vi "Gas Switching Menu Bar.vi"() -> ()   [LabVIEW 2015]
uses:
  <vilib>/Utility/miscctls.llb/LVRowAndColumnTypeDef.ctl
  <vilib>/Utility/file.llb/Read Delimited Spreadsheet (string).vi
panel:
  out "disabled index (col)":i32
  out "Color Box 2":u32(colorbox)
  out "Skip Current Row":bool
  out "Elapsed Time":dbl caption="Elapsed Time (s)"
  in  "stop":bool
  in  "Table Control":string[][](table)=[["1", "1", "13"], ["2", "3", "24"], ["3", "4", "31"], ["4", "2", "19"], ["5", "6", "11"], ["6", "8", "28"], ["7", "3", "17"], ["8", "4", "9"], ["9", "3", "14"], ["10", "7", "41"], ["11", "4", "27"], ["12", "2", "18"], ["13", "1", "19"], ["14", "7", "12"], ["15", "8", "28"], ["16", "5", "18"], ["17", "3", "27"], ["18", "2", "13"], ["19", "1", "31"], ["20", "6", "24"]]
  # "Auto Gas Switching"
  # "seconds"
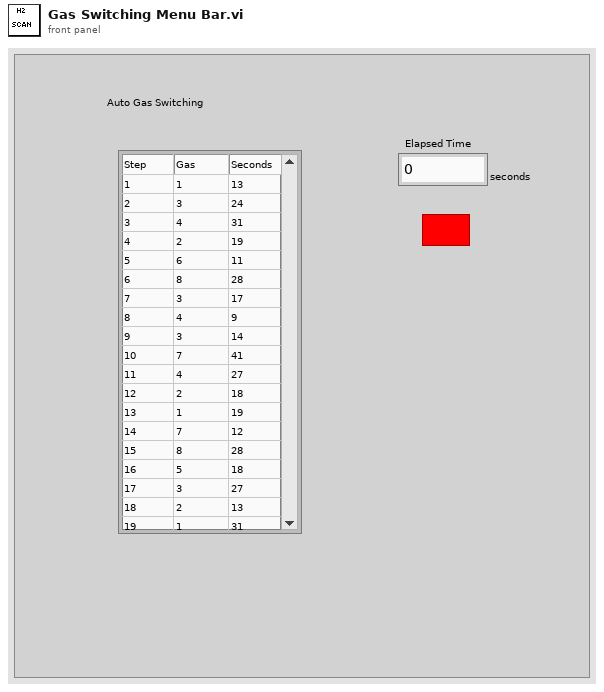
[diagram p1: front panel]
types:
  T1 = typedef "LVRowAndColumnTypeDef.ctl" = cluster{"Row":i32, "Column":i32}
  T2 = typedef "LVBoundsTypeDef.ctl" = cluster{"Width":u32, "Height":u32}
  T3 = typedef "LVPositionTypeDef.ctl" = cluster{"Left":i32, "Top":i32}
  T4 = typedef "LVPoint32TypeDef.ctl" = cluster{"Horizontal":i32, "Vertical":i32}
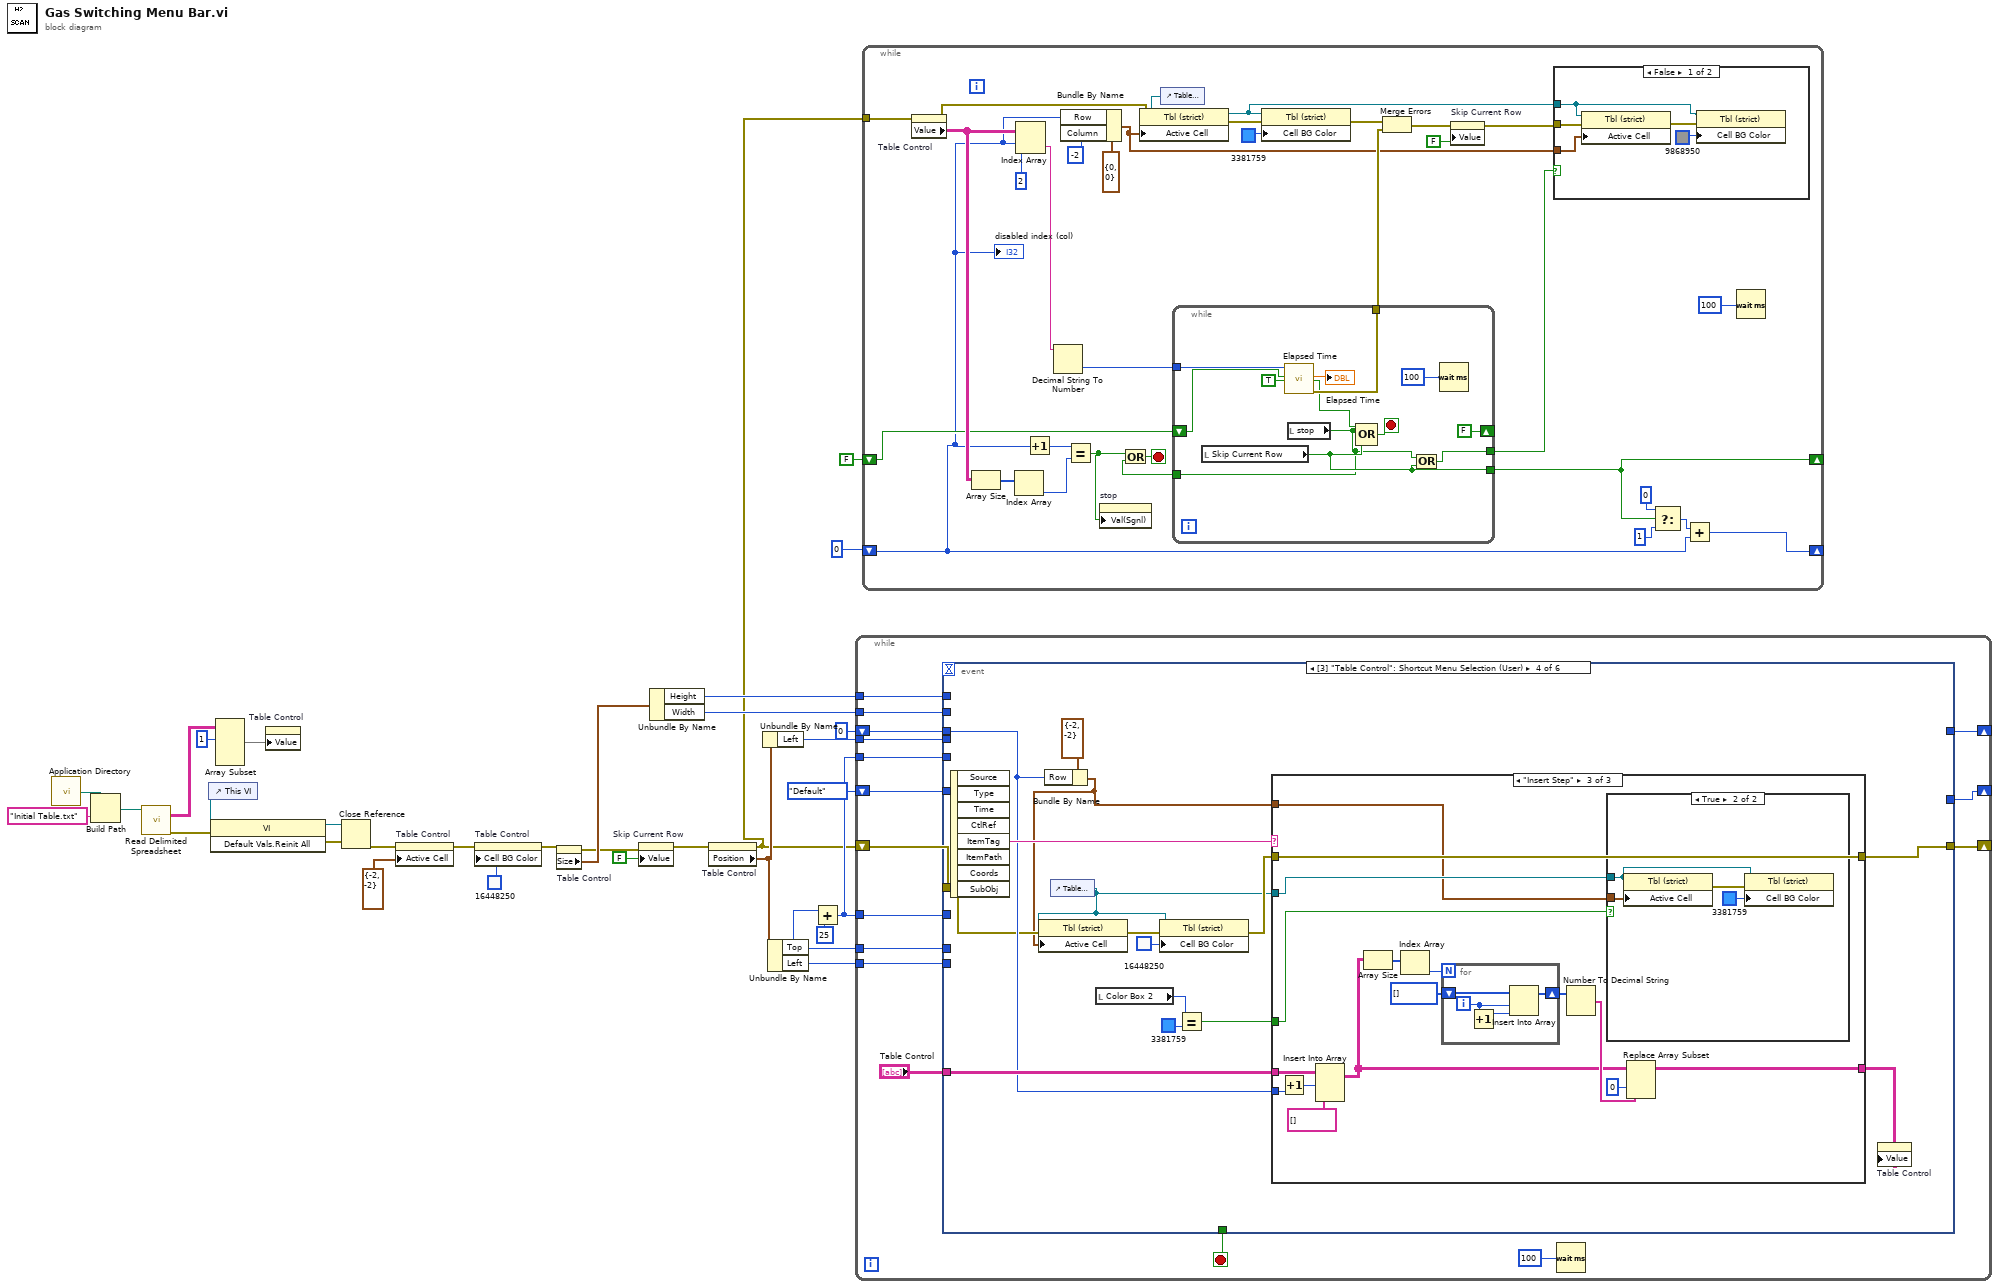
[diagram p0: block diagram]
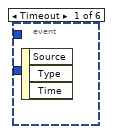
[diagram p3: hidden frame]
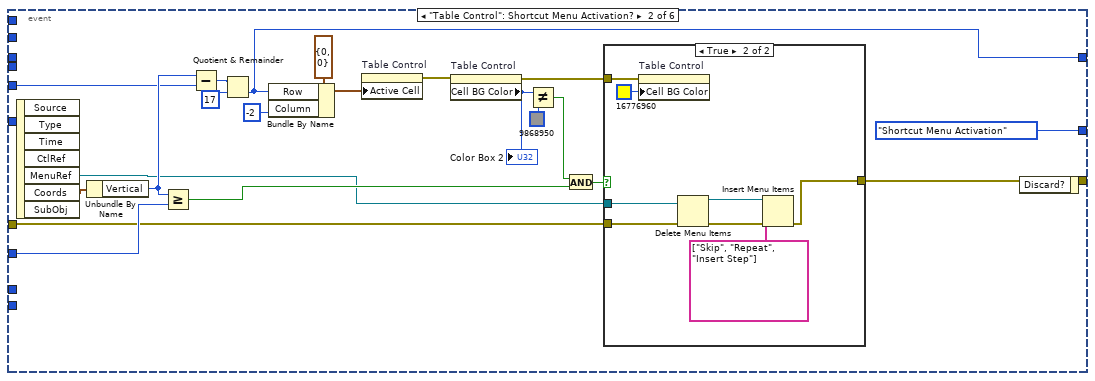
[diagram p4: hidden frame]
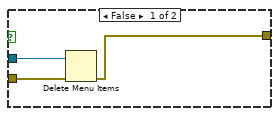
[diagram p5: hidden frame]
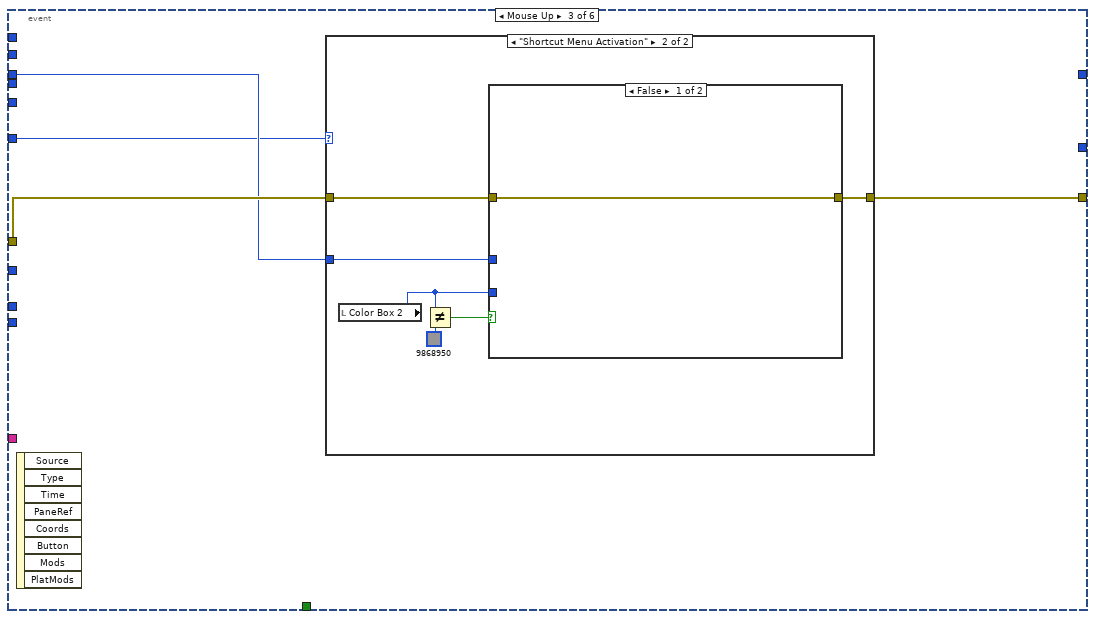
[diagram p6: hidden frame]
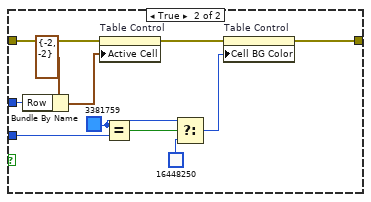
[diagram p8: hidden frame]
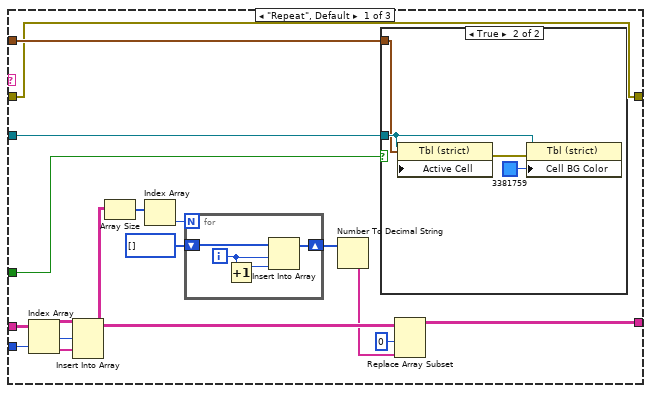
[diagram p9: hidden frame]
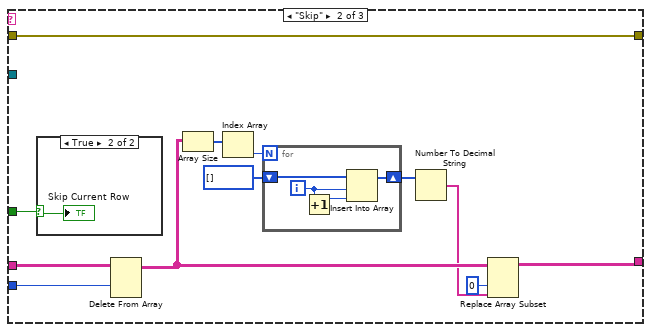
[diagram p11: hidden frame]
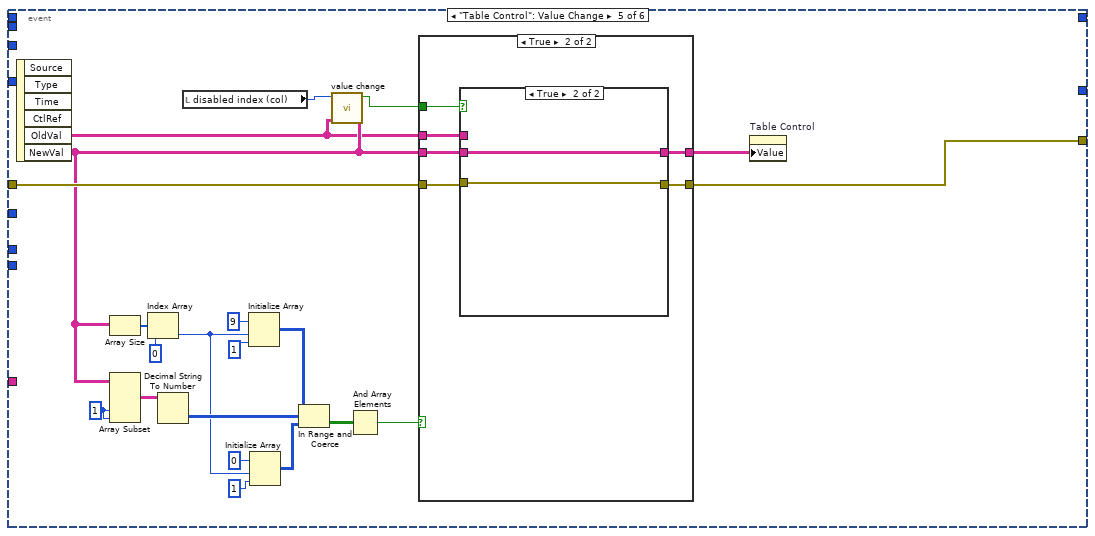
[diagram p14: hidden frame]
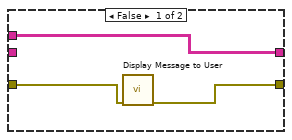
[diagram p15: hidden frame]
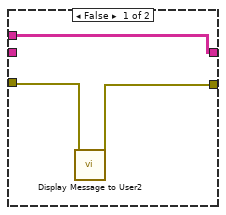
[diagram p16: hidden frame]
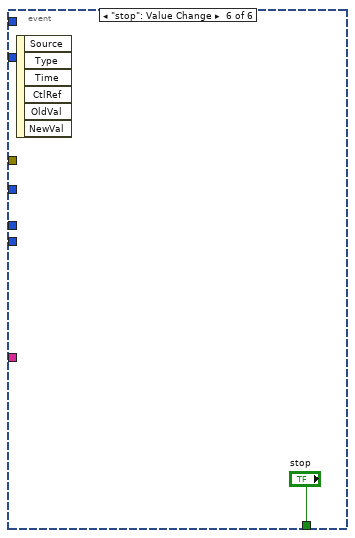
[diagram p17: hidden frame]
diagram:
  n1 = call <vilib>:"Application Directory.vi"() -> ("Application Directory"=w3:path)
  n2 = Build Path(base path=w3, name or relative path="Initial Table.txt") -> (appended path=w1:path)
  n3 = call-poly <vilib>:"Read Delimited Spreadsheet.vi"("file path (dialog if empty)"=w1) -> ("all rows"=w14:string[][], "error out"=w11:errorcluster)  [unwired: 9 in, 4 out]
  n4 = control-ref of="This VI"() -> (w30:refnum<vi>)
  n5 = invoke class="VI" method="Default Vals.Reinit All"(reference=w30, error in=w11) -> (reference out=w29:refnum<vi>, error out=w28:errorcluster)  [unwired: 1 in, 1 out]
  n6 = Array Subset(array=w14, index (row)=1 ("index")) -> (w12:string[][])  [unwired: 3 in]
  n7 = property on="Table Control" class="Tbl (strict)"("Value"=w12) -> ()  [unwired: 2 in, 2 out]
  n8 = Close Reference(reference=w29, error in (no error)=w28) -> (error out=w24:errorcluster)
  n9 = property on="Table Control" class="Tbl (strict)"(error in=w24, "Active Cell"=T1 {"Row"=-2, "Column"=-2} ("Active Cell:Active Cell")) -> (error out=w26:errorcluster)  [unwired: 1 in, 1 out]
  n10 = property on="Table Control" class="Tbl (strict)"(error in=w26, "Cell BG Color"=u32 16448250) -> (error out=w23:errorcluster)  [unwired: 1 in, 1 out]
  n11 = property on="Table Control" class="Tbl (strict)"(error in=w23) -> (error out=w8:errorcluster, "Size"=w21:T2)  [unwired: 1 in, 1 out]
  n12 = property on="Skip Current Row" class="Bool (strict)"(error in=w8, "Value"=FALSE ("Skip Current Row")) -> (error out=w7:errorcluster)  [unwired: 1 in, 1 out]
  n13 = Unbundle By Name(w21) -> ("Height"=w16:u32, "Width"=w20:u32)
  n14 = property on="Table Control" class="Tbl (strict)"(error in=w7) -> (error out=w10:errorcluster, "Position"=w19:T3)  [unwired: 1 in, 1 out]
  n15 = Unbundle By Name(w19) -> ("Left"=w18:i32)
  n16 = Unbundle By Name(w19) -> ("Top"=w17:i32, "Left"=w22:i32)
  n17 = Add(x=w17, y=25) -> (x+y=w31:i32)
  n18 = while {
    tunnel: w31 -> [w48]
    tunnel: w31 -> [w47]
    shift-right: [w46] -> _
    shift-left: w10 -> [w45]
    tunnel: w22 -> [w43]
    tunnel: w20 -> [w42]
    tunnel: w18 -> [w41]
    tunnel: w17 -> [w40]
    tunnel: w16 -> [w39]
    shift-right: [w38] -> _
    shift-left: 0 -> [w36]
    shift-right: [w35] -> _
    shift-left: enum16{"Default", "Shortcut Menu Activation"}."Default" -> [w34]
    stop <- w44 stop-if-true
    n19 = event shown="[3] \"Table Control\": Shortcut Menu Selection (User)" {
      selector: _ -> [_ _ _ _ _ _]
      dyn-events: _ -> [_ _ _ _ _ _]
      timeout: _ -> [_ _ _ _ _ _]
      tunnel: [_ _ _ _ _ "stop"] -> w44
      tunnel: w48 -> [_ w68 _ _ _ _]
      tunnel: w47 -> [_ w66 _ _ _ _]
      tunnel: [_ w50 w83 w107 w189 _] -> w46
      tunnel: w45 -> [_ w51 w84 w108 w187 _]
      tunnel: w43 -> [_ _ _ _ _ _]
      tunnel: w42 -> [_ _ _ _ _ _]
      tunnel: w41 -> [_ _ _ _ _ _]
      tunnel: w40 -> [_ _ _ _ _ _]
      tunnel: w39 -> [_ _ _ _ _ _]
      tunnel: [_ w64 _ _ _ _] -> w38
      tunnel: "Table Control" -> [_ _ _ w117 _ _]
      tunnel: w36 -> [_ _ w82 w113 _ _]
      tunnel: [_ enum16{"Default", "Shortcut Menu Activation"}."Shortcut Menu Activation" _ _ _ _] -> w35
      tunnel: w34 -> [_ _ w81 _ _ _]
      event Timeout {
        n20 = event-data() -> ()  [unwired: 1 in, 3 out]
      }
      event "Table Control": Shortcut Menu Activation? {
        n21 = event-data() -> ("MenuRef"=w52:refnum<k9>, "Coords"=w69:T4)  [unwired: 1 in, 5 out]
        n22 = Unbundle By Name(w69) -> ("Vertical"=w67:i32)
        n23 = Greater Or Equal?(x=w67, y=w68) -> (x >= y?=w55:bool)
        n24 = Subtract(x=w67, y=w66) -> (x-y=w65:i32)
        n25 = Quotient & Remainder(x=w65, y=17) -> (floor(x/y)=w64:i32)  [unwired: 1 out]
        n26 = Bundle By Name(cluster=T1 {"Row"=0, "Column"=0} ("Active Cell:Active Cell"), "Row"=w64, "Column"=-2) -> (w60:T1)
        n27 = property on="Table Control" class="Tbl (strict)"("Active Cell"=w60) -> (error out=w58:errorcluster)  [unwired: 2 in, 1 out]
        n28 = property on="Table Control" class="Tbl (strict)"(error in=w58) -> (error out=w53:errorcluster, "Cell BG Color"=w49:u32)  [unwired: 1 in, 1 out]
        "Color Box 2" <- w49
        n29 = Not Equal?(x=w49, y=u32 9868950) -> (x != y?=w56:bool)
        n30 = And(x=w56, y=w55) -> (x .and. y?=w54:bool)
        n31 = case shown="True" w54 {
          tunnel: w53 -> [_ w79]
          tunnel: w52 -> [w72 w75]
          tunnel: w51 -> [w71 w74]
          tunnel: [w70 w73] -> w50
          frame False {
            n32 = Delete Menu Items(6:w71, 9:w72) -> (0:w70:errorcluster)  [unwired: 2 in, 1 out]
          }
          frame True {
            n33 = property on="Table Control" class="Tbl (strict)"(error in=w79, "Cell BG Color"=u32 16776960) -> ()  [unwired: 1 in, 2 out]
            n34 = Delete Menu Items(6:w74, 9:w75) -> (0:w78:errorcluster, 3:w76:refnum<k9>)  [unwired: 2 in]
            n35 = Insert Menu Items(6:w78, 8:string[] ["Skip", "Repeat", "Insert Step"] ("item names"), 9:w76) -> (0:w73:errorcluster)  [unwired: 3 in, 2 out]
          }
        }
        n36 = event-data() -> ()  [unwired: 2 in, 1 out]
      }
      event Mouse Up {
        n37 = event-data() -> ()  [unwired: 1 in, 8 out]
        n38 = case shown="\"Shortcut Menu Activation\"" w81 {
          tunnel: w84 -> [w85 w91]
          tunnel: [w85 w90] -> w83
          tunnel: w82 -> [_ w89]
          frame "Default", Default {
          }
          frame "Shortcut Menu Activation" {
            n39 = local read "Color Box 2"() -> (w86:u32)
            n40 = Not Equal?(x=w86, y=u32 9868950) -> (x != y?=w87:bool)
            n41 = case shown="False" w87 {
              tunnel: w91 -> [w92 w102]
              tunnel: [w92 w101] -> w90
              tunnel: w89 -> [_ w100]
              tunnel: w86 -> [_ w96]
              frame False {
              }
              frame True {
                w95 = u32 3381759
                n42 = Bundle By Name(cluster=T1 {"Row"=-2, "Column"=-2} ("Active Cell:Active Cell"), "Row"=w100) -> (w98:T1)
                n43 = property on="Table Control" class="Tbl (strict)"(error in=w102, "Active Cell"=w98) -> (error out=w103:errorcluster)  [unwired: 1 in, 1 out]
                n44 = Equal?(x=w95, y=w96) -> (x = y?=w97:bool)
                n45 = Select(t=w95, s=w97, f=u32 16448250) -> (s? t:f=w93:u32)
                n46 = property on="Table Control" class="Tbl (strict)"(error in=w103, "Cell BG Color"=w93) -> (error out=w101:errorcluster)  [unwired: 1 in, 1 out]
              }
            }
          }
        }
      }
      event "Table Control": Shortcut Menu Selection (User) {
        n47 = event-data() -> ("ItemTag"=w118:string)  [unwired: 1 in, 7 out]
        n48 = Bundle By Name(cluster=T1 {"Row"=-2, "Column"=-2} ("Active Cell:Active Cell"), "Row"=w113) -> (w104:T1)
        n49 = control-ref of="Table Control"() -> (w105:refnum<vi>)
        n50 = property on="Property Node" class="Tbl (strict)"(reference=w105, error in=w108, "Active Cell"=w104) -> (error out=w116:errorcluster)  [unwired: 1 out]
        n51 = local read "Color Box 2"() -> (w106:u32)
        n52 = property on="Property Node" class="Tbl (strict)"(reference=w105, error in=w116, "Cell BG Color"=u32 16448250) -> (error out=w112:errorcluster)  [unwired: 1 out]
        n53 = Equal?(x=w106, y=u32 3381759) -> (x = y?=w109:bool)
        n54 = case shown="\"Insert Step\"" w118 {
          tunnel: w117 -> [w132 w153 w174]
          tunnel: w113 -> [w131 w152 w165]
          tunnel: [w123 w145 w166] -> w111
          tunnel: w112 -> [w119 w143 w162]
          tunnel: [w119 w143 w162] -> w107
          tunnel: w109 -> [w122 w142 w159]
          tunnel: w105 -> [w121 _ w161]
          tunnel: w104 -> [w120 _ w160]
          frame "Repeat", Default {
            n55 = Index Array(array=w132, index (row)=w131) -> (element=w133:string[])  [unwired: 1 in]
            n56 = Insert Into Array(array=w132, index (row)=w131, new element=w133) -> (w126:string[][])  [unwired: 1 in]
            n57 = Array Size(array=w126) -> (size(s)=w130:i32[])
            n58 = Index Array(array=w130) -> (element=w128:i32)  [unwired: 1 in]
            n59 = for {
              N: w128 -> [_]
              shift-right: [w139] -> w127
              shift-left: i32[] [] -> [w138]
              i -> [w141]
              n60 = Increment(x=w141) -> (x+1=w140:i32)
              n61 = Insert Into Array(array=w138, index=w141, new element=w140) -> (w139:i32[])
            }
            n62 = Number To Decimal String(number=w127) -> (decimal integer string=w125:string[])  [unwired: 1 in]
            n63 = case shown="True" w122 {
              tunnel: w121 -> [_ w136]
              tunnel: w120 -> [_ w135]
              frame False {
              }
              frame True {
                n64 = property on="Property Node" class="Tbl (strict)"(reference=w136, "Active Cell"=w135) -> (error out=w137:errorcluster)  [unwired: 1 in, 1 out]
                n65 = property on="Property Node" class="Tbl (strict)"(reference=w136, error in=w137, "Cell BG Color"=u32 3381759) -> ()  [unwired: 2 out]
              }
            }
            n66 = Replace Array Subset(array=w126, new element=w125, index (col)=0 ("disabled index (col)")) -> (w123:string[][])  [unwired: 1 in]
          }
          frame "Skip" {
            n67 = case shown="True" w142 {
              selector: w142 -> [_ w154]
              frame False {
              }
              frame True {
                "Skip Current Row" <- w154
              }
            }
            n68 = Delete From Array(array=w153, index (row)=w152) -> (array with subset deleted=w147:string[][])  [unwired: 2 in, 1 out]
            n69 = Array Size(array=w147) -> (size(s)=w151:i32[])
            n70 = Index Array(array=w151) -> (element=w149:i32)  [unwired: 1 in]
            n71 = for {
              N: w149 -> [_]
              shift-right: [w156] -> w148
              shift-left: i32[] [] -> [w155]
              i -> [w158]
              n72 = Increment(x=w158) -> (x+1=w157:i32)
              n73 = Insert Into Array(array=w155, index=w158, new element=w157) -> (w156:i32[])
            }
            n74 = Number To Decimal String(number=w148) -> (decimal integer string=w146:string[])  [unwired: 1 in]
            n75 = Replace Array Subset(array=w147, new element=w146, index (col)=0 ("disabled index (col)")) -> (w145:string[][])  [unwired: 1 in]
          }
          frame "Insert Step" {
            n76 = Increment(x=w165) -> (x+1=w164:i32)
            n77 = Insert Into Array(array=w174, index (row)=w164, new element=string[] [] ("new element/subarray")) -> (w167:string[][])  [unwired: 1 in]
            n78 = Array Size(array=w167) -> (size(s)=w173:i32[])
            n79 = Index Array(array=w173) -> (element=w171:i32)  [unwired: 1 in]
            n80 = for {
              N: w171 -> [_]
              shift-right: [w180] -> w170
              shift-left: i32[] [] -> [w179]
              i -> [w182]
              n81 = Increment(x=w182) -> (x+1=w181:i32)
              n82 = Insert Into Array(array=w179, index=w182, new element=w181) -> (w180:i32[])
            }
            n83 = Number To Decimal String(number=w170) -> (decimal integer string=w169:string[])  [unwired: 1 in]
            n84 = case shown="True" w159 {
              tunnel: w161 -> [_ w176]
              tunnel: w160 -> [_ w175]
              frame False {
              }
              frame True {
                n85 = property on="Property Node" class="Tbl (strict)"(reference=w176, "Active Cell"=w175) -> (error out=w178:errorcluster)  [unwired: 1 in, 1 out]
                n86 = property on="Property Node" class="Tbl (strict)"(reference=w176, error in=w178, "Cell BG Color"=u32 3381759) -> ()  [unwired: 2 out]
              }
            }
            n87 = Replace Array Subset(array=w167, new element=w169, index (col)=0 ("disabled index (col)")) -> (w166:string[][])  [unwired: 1 in]
          }
        }
        n88 = property on="Table Control" class="Tbl (strict)"("Value"=w111) -> ()  [unwired: 2 in, 2 out]
      }
      event "Table Control": Value Change {
        w203 = 1 ("index")
        n89 = event-data() -> ("OldVal"=w184:string[][], "NewVal"=w185:string[][])  [unwired: 1 in, 4 out]
        n90 = Array Size(array=w185) -> (size(s)=w200:i32[])
        n91 = Array Subset(array=w185, index (col)=w203, length (col)=w203) -> (w202:string[][])  [unwired: 2 in]
        n92 = Index Array(array=w200, index=0) -> (element=w194:i32)
        n93 = Decimal String To Number(string=w202) -> (number=w201:i32[][])  [unwired: 2 in, 1 out]
        n94 = local read "disabled index (col)"() -> (w183:i32)
        n95 = Initialize Array(9 ("index"), w194, 1 ("dimension size")) -> (w188:i32[][])
        n96 = Initialize Array(0 ("index"), w194, 1 ("dimension size")) -> (w193:i32[][])
        n97 = In Range and Coerce(upper limit=w188, x=w201, lower limit=w193) -> (In Range?=w192:bool[][])  [unwired: 1 out]
        n98 = call "value change.vi"("NewVal"=w185, "OldVal"=w184, "disabled index (col)"=w183) -> ("x > y?"=w186:bool)  [unwired: 8 in]
        n99 = And Array Elements(Boolean array=w192) -> (logical AND=w191:bool)
        n100 = case shown="True" w191 {
          tunnel: [w206 w210] -> w190
          tunnel: w185 -> [_ w208]
          tunnel: w184 -> [w206 w209]
          tunnel: w187 -> [w205 w212]
          tunnel: [w204 w211] -> w189
          tunnel: w186 -> [_ w207]
          frame False {
            n101 = call "Display Message to User"("error in (no error)"=w205) -> ("error out"=w204:errorcluster)  [unwired: 9 in, 1 out]
          }
          frame True {
            n102 = case shown="True" w207 {
              tunnel: w212 -> [w215 w217]
              tunnel: [w214 w217] -> w211
              tunnel: [w213 w216] -> w210
              tunnel: w209 -> [w213 _]
              tunnel: w208 -> [_ w216]
              frame False {
                n103 = call "Display Message to User2"("error in (no error)"=w215) -> ("error out"=w214:errorcluster)  [unwired: 9 in, 1 out]
              }
              frame True {
              }
            }
          }
        }
        n104 = property on="Table Control" class="Tbl (strict)"("Value"=w190) -> ()  [unwired: 2 in, 2 out]
      }
      event "stop": Value Change {
        n105 = event-data() -> ()  [unwired: 1 in, 6 out]
      }
    }
    n106 = Wait (ms)(milliseconds to wait=u32 100 ("millisecond timer value")) -> ()  [unwired: 1 out]
  }
  n107 = while {
    tunnel: w10 -> [w243]
    shift-right: [w223] -> _
    shift-left: FALSE ("Skip Current Row") -> [w229]
    shift-right: [w222] -> _
    shift-left: 0 ("disabled index (col)") -> [w221]
    stop <- w246 stop-if-true
    n108 = property on="Table Control" class="Tbl (strict)"(error in=w243) -> (error out=w237:errorcluster, "Value"=w249:string[][])  [unwired: 1 in, 1 out]
    n109 = Array Size(array=w249) -> (size(s)=w250:i32[])
    n110 = Index Array(array=w250) -> (element=w245:i32)  [unwired: 1 in]
    n111 = Index Array(array=w249, index (row)=w221, index (col)=2 ("disabled index (col)")) -> (element=w247:string)
    n112 = Increment(x=w221) -> (x+1=w244:i32)
    n113 = Decimal String To Number(string=w247) -> (number=w248:i32)  [unwired: 2 in, 1 out]
    n114 = Bundle By Name(cluster=T1 {"Row"=0, "Column"=0} ("Active Cell:Active Cell"), "Row"=w221, "Column"=-2) -> (w234:T1)
    n115 = Equal?(x=w244, y=w245) -> (x = y?=w220:bool)
    n116 = property on="stop" class="Bool (strict)"("Val(Sgnl)"=w220) -> ()  [unwired: 2 in, 2 out]
    n117 = control-ref of="Table Control"() -> (w233:refnum<vi>)
    n118 = property on="Property Node" class="Tbl (strict)"(reference=w233, error in=w237, "Active Cell"=w234) -> (error out=w242:errorcluster)  [unwired: 1 out]
    n119 = while {
      tunnel: w248 -> [w267]
      tunnel: [w264] -> w235
      tunnel: [w257] -> w228
      tunnel: [w258] -> w223
      shift-right: [FALSE ("Skip Current Row")] -> _
      shift-left: w229 -> [w262]
      tunnel: [w256] -> w227
      stop <- w263 stop-if-true
      n120 = local read "Skip Current Row"() -> (w258:bool)
      n121 = call "Elapsed Time"("Time Target (s)"=w267, "Reset"=w262, "Auto Reset"=TRUE) -> ("Elapsed Time (s)"=→"Elapsed Time":dbl, "Time has Elapsed"=w259:bool, "error out"=w264:errorcluster)  [unwired: 9 in, 5 out]
      n122 = local read "stop"() -> (w256:bool)
      n123 = Compound Arithmetic op=OR(w259, w256, w258) -> (w263:bool)
      n124 = Or(x=w256, y=w258) -> (x .or. y?=w257:bool)
      n125 = Wait (ms)(milliseconds to wait=u32 100 ("millisecond timer value")) -> ()  [unwired: 1 out]
    }
    n126 = Or(x=w220, y=w227) -> (x .or. y?=w246:bool)
    n127 = property on="Property Node" class="Tbl (strict)"(reference=w233, error in=w242, "Cell BG Color"=u32 3381759) -> (error out=w236:errorcluster)  [unwired: 1 out]
    n128 = Merge Errors(w236, w235) -> (w231:errorcluster)
    n129 = property on="Skip Current Row" class="Bool (strict)"(error in=w231, "Value"=FALSE ("Skip Current Row")) -> (error out=w230:errorcluster)  [unwired: 1 in, 1 out]
    n130 = case shown="False" w228 {
      tunnel: w230 -> [w253 _]
      tunnel: w234 -> [w252 _]
      tunnel: w233 -> [w251 _]
      frame False {
        n131 = property on="Property Node" class="Tbl (strict)"(reference=w251, error in=w253, "Active Cell"=w252) -> (error out=w254:errorcluster)  [unwired: 1 out]
        n132 = property on="Property Node" class="Tbl (strict)"(reference=w251, error in=w254, "Cell BG Color"=u32 9868950) -> ()  [unwired: 2 out]
      }
      frame True {
      }
    }
    n133 = Select(t=0 ("disabled index (col)"), s=w223, f=1 ("disabled index (col)")) -> (s? t:f=w224:i32)
    n134 = Add(x=w224, y=w221) -> (x+y=w222:i32)
    n135 = Wait (ms)(milliseconds to wait=u32 100 ("millisecond timer value")) -> ()  [unwired: 1 out]
    "disabled index (col)" <- w221
  }
